vi "ObjectHandler.GetCycleRefs.vi"(8 "error in (no error)":errorcluster, 11 "ObjectHandler in":refnum<class "ObjectHandler.lvclass">) -> (0 "error out":errorcluster, 2 "ObjectArray":T1[](array[typedef]), 3 "ObjectHandler out":refnum<class "ObjectHandler.lvclass">)   [LabVIEW 2016, in "ObjectHandler.lvclass"]
uses:
  ObjectHandler.lvclass
  ObjectHandler.ObjectWType.ctl
  ObjectHandler.ObjectType.ctl
  ObjectHandler.lvclass/ObjectHandler.ctl
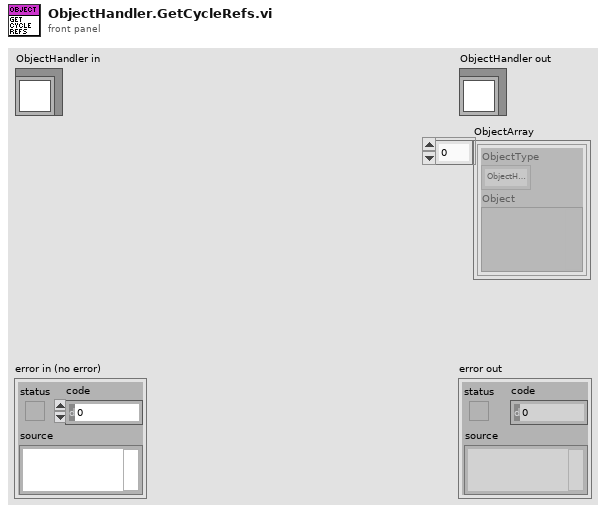
[diagram p1: front panel]
types:
  T1 = typedef "ObjectHandler.lvclass/ObjectHandler.ObjectWType.ctl" = cluster{"ObjectType":T2, "Object":variant}
  T2 = typedef "ObjectHandler.lvclass/ObjectHandler.ObjectType.ctl" = enum16{"undefined", "ObjectHandler", "ViHandler", "ErrorHandler", "CentralStorage", "Hausmodell", "Sondenmodell", "Wärmepumpe", "Umgebung"}
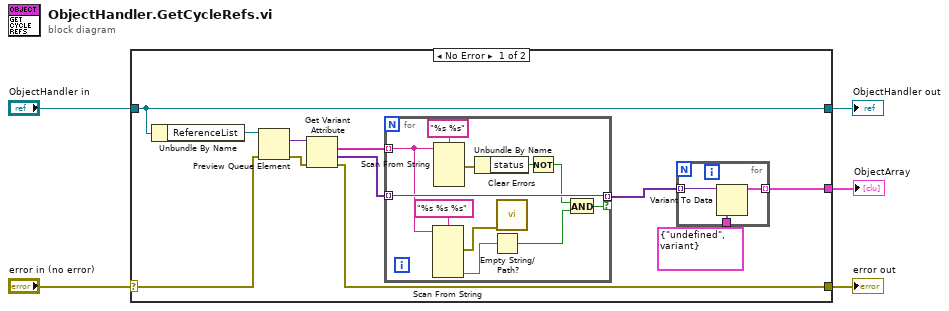
[diagram p0: block diagram]
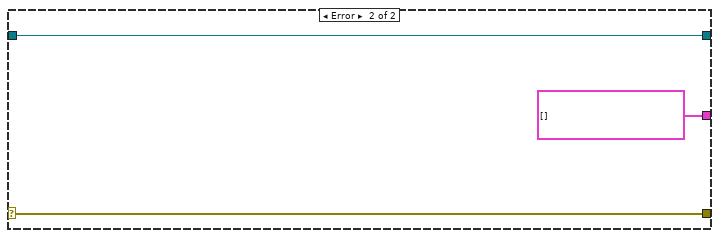
[diagram p2: hidden frame]
diagram:
  n1 = case shown="No Error" "error in (no error)" {
    selector: "error in (no error)" -> [w12 w33]
    tunnel: [w11 w33] -> w4
    tunnel: [w16 w32] -> w2
    tunnel: "ObjectHandler in" -> [w16 w32]
    tunnel: [w6 T1[] [] ("ObjectArray")] -> w1
    frame No Error {
      n2 = Unbundle By Name(w16) -> ("ReferenceList"=w15:refnum<queue>)
      n3 = Preview Queue Element(queue=w15, error in (no error)=w12) -> (element=w14:variant, error out=w13:errorcluster)  [unwired: 1 in, 2 out]
      n4 = Get Variant Attribute(Variant=w14, error in=w13) -> (names=w10:string[], values=w9:variant[], error out=w11:errorcluster)  [unwired: 2 in, 1 out]
      n5 = for {
        tunnel: w10 -> [w27] mode=indexing
        tunnel: w9 -> [w28] mode=indexing
        tunnel: [w28] -> w7 mode=indexing if=w21
        n6 = Scan From String(format string="%s %s %s", input string=w27) -> (error out=w20:errorcluster, output 3=w25:string)  [unwired: 7 in, 2 out]
        n7 = Scan From String(format string="%s %s", input string=w27) -> (error out=w29:errorcluster)  [unwired: 6 in, 2 out]
        n8 = Unbundle By Name(w29) -> ("status"=w23:bool)
        n9 = Empty String/Path?(string/path=w25) -> (empty?=w22:bool)
        n10 = call <vilib>:"Clear Errors.vi"("error in (no error)"=w20) -> ()  [unwired: 5 in, 2 out]
        n11 = Not(x=w23) -> (.not. x?=w24:bool)
        n12 = And(x=w24, y=w22) -> (x .and. y?=w21:bool)
      }
      n13 = for {
        tunnel: w7 -> [w19] mode=indexing
        tunnel: T1 {"ObjectType"=enum."undefined", "Object"=variant} ("ObjectWType") -> [w18]
        tunnel: [w17] -> w6 mode=indexing
        n14 = Variant To Data(type=w18, Variant=w19) -> (data=w17:T1)  [unwired: 1 in, 1 out]
      }
    }
    frame Error {
    }
  }
  "error out" <- w4
  "ObjectHandler out" <- w2
  "ObjectArray" <- w1
